vi "ComplexStringToComplexNumber.vi"(11 "String":string) -> (3 "Numeric":cdb)   [LabVIEW 2014, in "Visualization.lvlib" / "VisualizeAppLSE.lvclass"]
uses:
  VisualizeAppLSE.lvclass
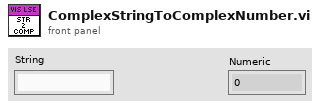
[diagram p1: front panel]
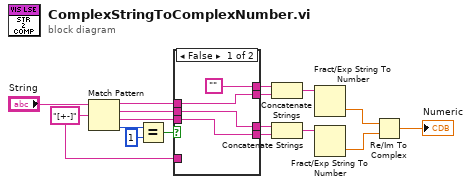
[diagram p0: block diagram]
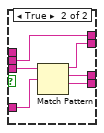
[diagram p2: hidden frame]
diagram:
  w9 = "[+-]" ("regular expression")
  n1 = Match Pattern(string="String", regular expression=w9) -> (before substring=w8:string, match substring=w7:string, after substring=w10:string, offset past match=w13:i32)  [unwired: 1 in]
  n2 = Equal?(x=w13, y=1) -> (x = y?=w11:bool)
  n3 = case shown="False" w11 {
    tunnel: w10 -> [w21 w27]
    tunnel: w9 -> [_ w26]
    tunnel: [w20 w25] -> w3
    tunnel: [w21 w24] -> w4
    tunnel: w8 -> [w20 _]
    tunnel: w7 -> [w19 w22]
    tunnel: [w19 w23] -> w5
    tunnel: ["" w22] -> w2
    frame False {
    }
    frame True {
      n4 = Match Pattern(string=w27, regular expression=w26) -> (before substring=w25:string, match substring=w23:string, after substring=w24:string)  [unwired: 1 in, 1 out]
    }
  }
  n5 = Concatenate Strings(w2, w3) -> (w1:string)
  n6 = Concatenate Strings(w5, w4) -> (w6:string)
  n7 = Fract/Exp String To Number(string=w1) -> (number=w16:dbl)  [unwired: 3 in, 1 out]
  n8 = Fract/Exp String To Number(string=w6) -> (number=w15:dbl)  [unwired: 3 in, 1 out]
  n9 = Re/Im To Complex(1:w15, 2:w16) -> (0:→"Numeric":cdb)
